vi "HAL_Close.vi"(8 "error in":errorcluster, 11 "Handle In":T1) -> (0 "error out":errorcluster)   [LabVIEW 2015]
uses:
  Handle.ctl
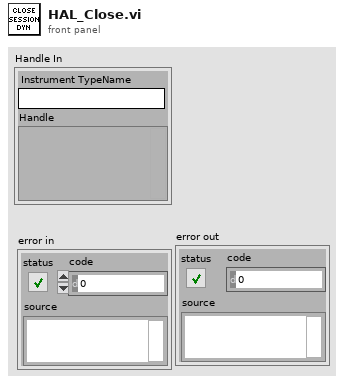
[diagram p1: front panel]
types:
  T1 = typedef "Handle.ctl" = cluster{"Instrument TypeName":string, "Handle":variant}
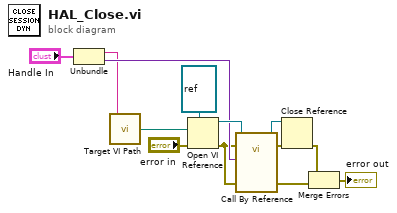
[diagram p0: block diagram]
diagram:
  n1 = Unbundle("Handle In") -> ("Instrument TypeName"=w6:string, "Handle"=w11:variant)
  n2 = call "Target VI Path.vi"("Instrument Name"=w6) -> ("Path to VI"=w7:path)
  n3 = Open VI Reference(type specifier VI Refnum (for type only)=refnum<vi> refnum, vi path=w7, error in (no error)="error in") -> (vi reference=w12:refnum<vi>, error out=w4:errorcluster)  [unwired: 3 in]
  n4 = call-by-ref "?"(reference=w12, error in=w4, "error in"=w4, "Handle"=w11) -> (reference out=w3:refnum<vi>, error out=w2:errorcluster, 0:"error out"=w9:errorcluster)  [unwired: 9 in]
  n5 = Close Reference(reference=w3, error in (no error)=w2) -> (error out=w1:errorcluster)
  n6 = Merge Errors(w1, w9) -> (→"error out":errorcluster)
